vi "Actor Core.vi"(8 "error in":errorcluster, 11 "_Parent Actor Template in":refnum<class "_Parent Actor Template.lvclass">) -> (0 "error out":errorcluster, 3 "Actor out":refnum<class "Actor.lvclass">)   [LabVIEW 2016, in "_Parent Actor Template.lvlib" / "_Parent Actor Template.lvclass"]
doc: "(<B>Filename</B>: Actor Framework.lvlib:Actor.lvclass:Actor Core.vi)\n\nReceives messages to the actor, reacts to them, and initiates any error handling that may shut the actor down.\n\nDescendant classes may override this VI to append parallel tasks for the actor to complete while it handles messages. Overrides use the Call Parent Method node."
uses:
  _Parent Actor Template.lvclass
  <vilib>/ActorFramework/Actor/Actor.lvclass
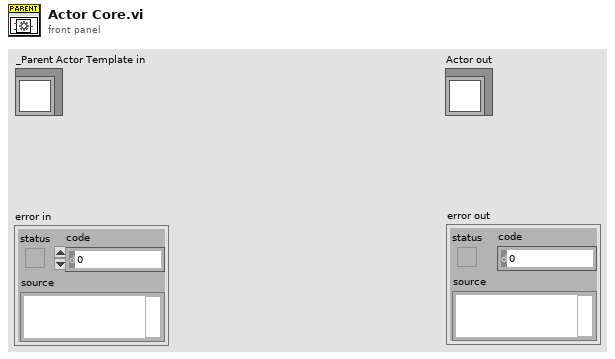
[diagram p1: front panel]
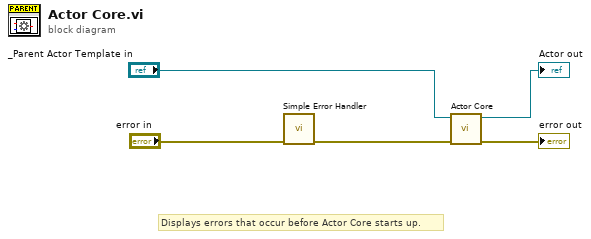
[diagram p0: block diagram]
diagram:
  # "Displays errors that occur before Actor Core starts up."
  n1 = call <vilib>:"Simple Error Handler.vi"("error in (no error)"="error in") -> ("error out"=w1:errorcluster)  [unwired: 4 in, 4 out]
  n2 = call-parent "Actor Core.vi"("error in"=w1, "Actor in"="_Parent Actor Template in") -> ("error out"=→"error out":errorcluster, "Actor out"=→"Actor out":refnum<class "Actor.lvclass">)  [unwired: 8 in]
